vi "Global 1.vi"() -> ()   [LabVIEW 2017]
panel:
  in  "Alliance":string
  in  "GameD":string
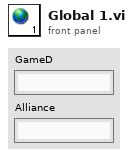
[diagram p1: front panel]
diagram:
